vi "Close Process Session.vi"(8 "error in (no error)":errorcluster, 11 "session ID":i32 format="%.0x") -> (0 "error out":errorcluster)   [LabVIEW 2013]
uses:
  ProcessSession.dll
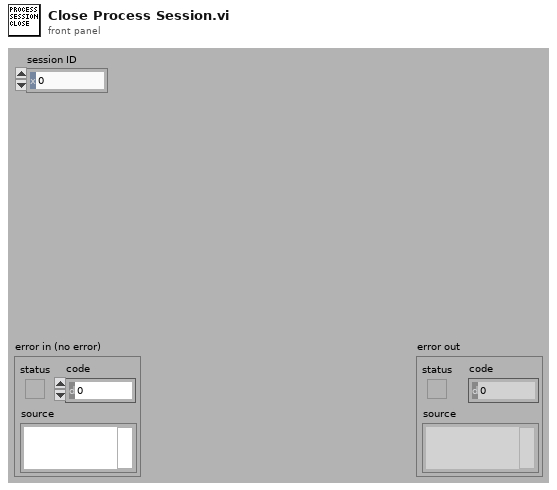
[diagram p1: front panel]
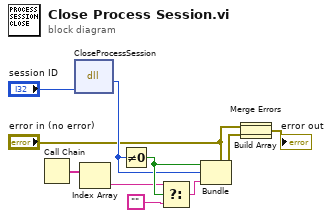
[diagram p0: block diagram]
diagram:
  n1 = Call Chain() -> (call chain=w8:string[])
  n2 = dll-call lib="C:/Users/inghoshr/Documents/LabVIEW Data/SmoketestVMVi/Process Session/ProcessSession.dll" fn="CloseProcessSession"("session"="session ID") -> (w5:i32)  [unwired: 4 in, 2 out]
  n3 = Index Array(array=w8) -> (element=w7:string)  [unwired: 1 in]
  n4 = Not Equal To 0?(x=w5) -> (x != 0?=w11:bool)
  n5 = Select(t=w7, s=w11, f="") -> (s? t:f=w9:string)
  n6 = Bundle(cluster="error in (no error)", "status"=w11, "code"=w5, "source"=w9) -> (w3:errorcluster)
  n7 = Build Array("error in (no error)", w3) -> (w1:errorcluster[])
  n8 = Merge Errors(w1) -> (→"error out":errorcluster)
